vi "SetRunMode.vi"(8 "error in (no error)":errorcluster, 10 "RunMode":T1, 11 "ScopeBase in":refnum<class "ScopeBase.lvclass">) -> (0 "error out":errorcluster, 3 "ScopeBase out":refnum<class "ScopeBase.lvclass">)   [LabVIEW 2018, in "ScopeBase.lvclass"]
uses:
  ScopeBase.lvclass
  controls/ScopeMode.ctl
  ScopeBase.lvclass/ScopeBase.ctl
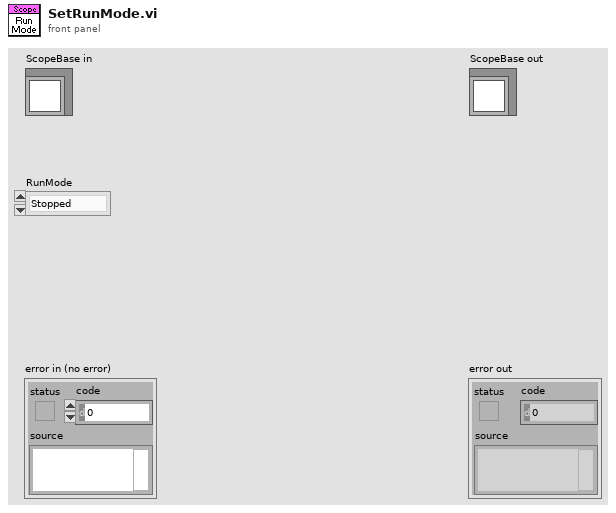
[diagram p1: front panel]
types:
  T1 = typedef "ScopeMode.ctl" = enum16{"Stopped", "Single", "Running", "Continuous"}
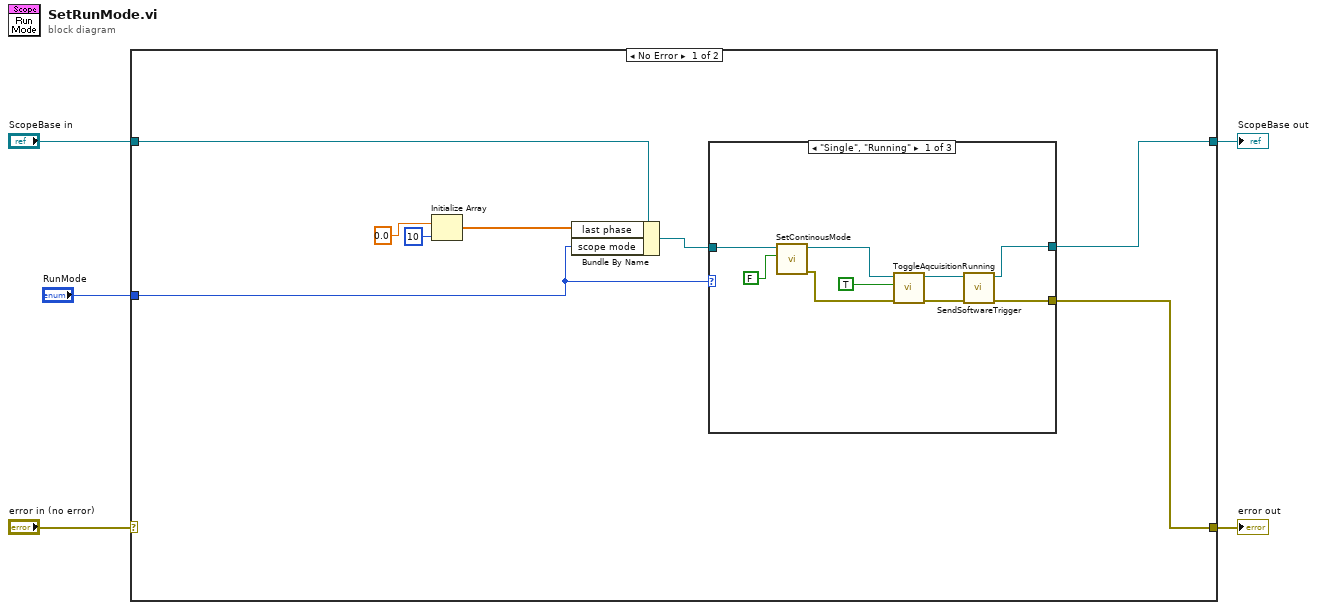
[diagram p0: block diagram]
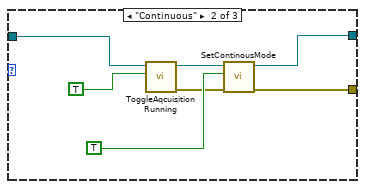
[diagram p2: hidden frame]
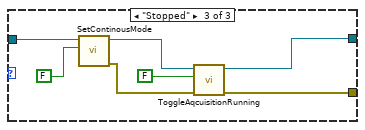
[diagram p3: hidden frame]
diagram:
  n1 = case shown="No Error" "error in (no error)" {
    selector: "error in (no error)" -> [_ w38]
    tunnel: [w9 w38] -> w4
    tunnel: [w11 w37] -> w2
    tunnel: "ScopeBase in" -> [w12 w37]
    tunnel: "RunMode" -> [w10 _]
    frame No Error {
      n2 = Initialize Array(0.0, 10 ("dimension size")) -> (w6:dbl[])
      n3 = Bundle By Name(cluster=w12, "last phase"=w6, "scope mode"=w10) -> (w13:refnum<class "ScopeBase.lvclass">)
      n4 = case shown="\"Single\", \"Running\"" w10 {
        tunnel: w13 -> [w19 w26 w33]
        tunnel: [w17 w28 w35] -> w11
        tunnel: [w14 w23 w30] -> w9
        frame "Single", "Running" {
          n5 = call-dynamic "SetContinousMode.vi"("Cont Acquisition"=FALSE, "ScopeBase In"=w19) -> ("error out"=w16:errorcluster, "ScopeBase Out"=w20:refnum<class "ScopeBase.lvclass">)  [unwired: 8 in]
          n6 = call-dynamic "ToggleAqcuisitionRunning.vi"("error in (no error)"=w16, "Acquisition running"=TRUE, "ScopeBase In"=w20) -> ("error out"=w15:errorcluster, "ScopeBase Out"=w18:refnum<class "ScopeBase.lvclass">)  [unwired: 7 in]
          n7 = call-dynamic "SendSoftwareTrigger.vi"("error in (no error)"=w15, "ScopeBase In"=w18) -> ("error out"=w14:errorcluster, "ScopeBase Out"=w17:refnum<class "ScopeBase.lvclass">)  [unwired: 8 in]
        }
        frame "Continuous" {
          n8 = call-dynamic "ToggleAqcuisitionRunning.vi"("Acquisition running"=TRUE, "ScopeBase In"=w26) -> ("error out"=w24:errorcluster, "ScopeBase Out"=w25:refnum<class "ScopeBase.lvclass">)  [unwired: 8 in]
          n9 = call-dynamic "SetContinousMode.vi"("error in (no error)"=w24, "Cont Acquisition"=TRUE ("Acquisition running"), "ScopeBase In"=w25) -> ("error out"=w23:errorcluster, "ScopeBase Out"=w28:refnum<class "ScopeBase.lvclass">)  [unwired: 7 in]
        }
        frame "Stopped" {
          n10 = call-dynamic "SetContinousMode.vi"("Cont Acquisition"=FALSE, "ScopeBase In"=w33) -> ("error out"=w31:errorcluster, "ScopeBase Out"=w32:refnum<class "ScopeBase.lvclass">)  [unwired: 8 in]
          n11 = call-dynamic "ToggleAqcuisitionRunning.vi"("error in (no error)"=w31, "Acquisition running"=FALSE, "ScopeBase In"=w32) -> ("error out"=w30:errorcluster, "ScopeBase Out"=w35:refnum<class "ScopeBase.lvclass">)  [unwired: 7 in]
        }
      }
    }
    frame Error {
    }
  }
  "error out" <- w4
  "ScopeBase out" <- w2
